vi "CAN_Float_Write_Example.vi"() -> ()   [LabVIEW 2019]
panel:
  in  "writeValue":sgl
  in  "SubIndex":i32=1 format="%x"
  in  "Index":i32=8194 format="%x"
  in  "CAN Module\nNode ID":i32=3
  in  "Instrument Type":i32(ring)=2 items=["PPMS", "VersaLab", "DynaCool", "SVSM", "OptiCool"]
  in  "Remote":bool
  in  "IP Address":string="127.0.0.1"
  # "Instrument Connection"
  # "Float SDO Write"
  # "2002.1 is adjustable module time"
  # "Node 3 is TCM. Pick a node that is present in your system for this test."
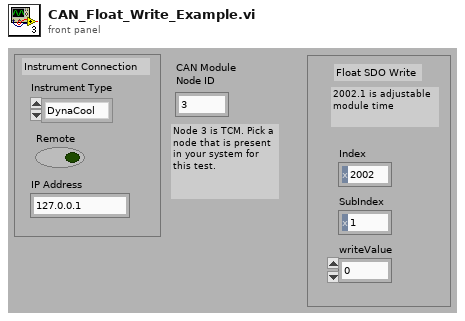
[diagram p1: front panel]
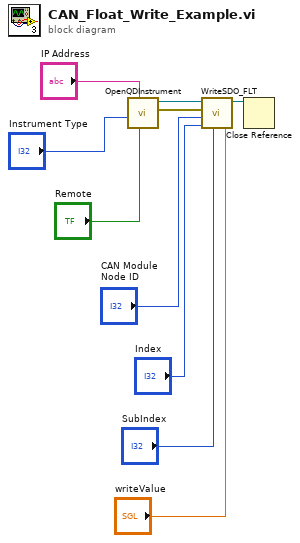
[diagram p0: block diagram]
diagram:
  n1 = call "OpenQDInstrument.vi"("Remote"="Remote", "IP Address"="IP Address", "InstrumentType"="Instrument Type") -> ("error out"=w9:errorcluster, "Instrument Ref"=w10:refnum<k24>)  [unwired: 5 in]
  n2 = call "WriteSDO_FLT.vi"("writeValue"="writeValue", "SubIndex"="SubIndex", "Index"="Index", "nodeID"="CAN Module\nNode ID", "error in (no error)"=w9, "Instrument Ref In"=w10) -> ("Instrument Ref Out"=w2:refnum<k24>)  [unwired: 2 in, 1 out]
  n3 = Close Reference(reference=w2) -> ()  [unwired: 1 in, 1 out]
